vi "Navigation_Main_r1.5 (going back to derp).vi"() -> ()   [LabVIEW 2015]
uses:
  <vilib>/myRIO/Instrument Drivers/Onboard IO/PWM/typedefs/PWM Reference.ctl
  <vilib>/myRIO/Common/Instrument Driver Framework/Utilities/typedefs/myRIO Generic Hardware Reference.ctl
  <vilib>/myRIO/Common/Instrument Driver Framework/Utilities/typedefs/Hardware Version Enum.ctl
  <vilib>/myRIO/Common/Instrument Driver Framework/Utilities/typedefs/myRIO v1.0 Reference.ctl
  <vilib>/myRIO/Common/Instrument Driver Framework/Utilities/typedefs/Generic FPGA Reference.ctl
  <vilib>/myRIO/Common/Instrument Driver Framework/myRIO v1.0/PWM/typedefs/PWM Channels Enum.ctl
  <vilib>/myRIO/Instrument Drivers/Onboard IO/PWM/typedefs/PWM Configuration.ctl
  <vilib>/userdefined/High Color/nirio_resource_hc.ctl
  <vilib>/myRIO/Common/Instrument Driver Framework/myRIO v1.0/PWM/vis/myRIO v1.1 Open PWM.vi
  <vilib>/myRIO/Common/Instrument Driver Framework/Utilities/vis/Validate Channels.vi
  <vilib>/myRIO/Common/Instrument Driver Framework/myRIO v1.0/PWM/vis/myRIO v1.0 Reserve PWM.vi
  <vilib>/myRIO/Common/Instrument Driver Framework/myRIO v1.0/PWM/vis/myRIO v1.0 Close PWM.vi
  <vilib>/myRIO/Common/Instrument Driver Framework/myRIO v1.0/PWM/vis/myRIO v1.0 Build MUX Configuration PWM.vi
  <vilib>/myRIO/Common/Instrument Driver Framework/myRIO v1.0/Resource Manager/vis/myRIO v1.0 Reserve Channel List.vi
  <vilib>/myRIO/Common/Instrument Driver Framework/myRIO v1.0/PWM/vis/myRIO v1.0 Unreserve PWM.vi
  <vilib>/myRIO/Common/Instrument Driver Framework/myRIO v1.0/Resource Manager/vis/myRIO v1.0 Create Configuration List.vi
  <vilib>/myRIO/Common/Instrument Driver Framework/myRIO v1.0/Resource Manager/vis/myRIO v1.0 Reserve Channel.vi
  <vilib>/myRIO/Common/Instrument Driver Framework/myRIO v1.0/Resource Manager/vis/myRIO v1.0 Unreserve Channel.vi
  <vilib>/myRIO/Common/Instrument Driver Framework/myRIO v1.0/Resource Manager/vis/myRIO v1.0 Unreserve Channel List.vi
  <vilib>/myRIO/Common/Instrument Driver Framework/myRIO v1.0/Resource Manager/vis/myRIO v1.0 Build Mutex Name.vi
  <vilib>/FPGAPlugInAG/myRIO-1900/niLvFpga_Open_myRIO-1900.vi
  <vilib>/rvi/interface/common/dynamic/niFpgaDynamicAddResources.vi
  <vilib>/myRIO/Common/Instrument Driver Framework/Utilities/vis/FPGA Ref Manager.vi
  <vilib>/Utility/error.llb/Error Cluster From Error Code.vi
  <vilib>/myRIO/Common/Instrument Driver Framework/Utilities/vis/Ref Counter.vi
  <vilib>/rvi/errors/niLvFpgaAdjustHostInterfaceError.vi
  <vilib>/Utility/VariantDataType/GetNumericInfo.vi
  <vilib>/myRIO/Common/Instrument Driver Framework/myRIO v1.0/myRIO v1.1 Open.vi
  <vilib>/myRIO/Common/Instrument Driver Framework/Utilities/vis/IO Manager.vi
  <vilib>/myRIO/Common/Instrument Driver Framework/Utilities/vis/Configuration Manager.vi
  <vilib>/myRIO/Common/Instrument Driver Framework/myRIO v1.0/Resource Manager/vis/myRIO v1.0 Configure IO.vi
  <vilib>/myRIO/Common/Instrument Driver Framework/myRIO v1.0/myRIO v1.0 Close.vi
  <vilib>/myRIO/Common/Instrument Driver Framework/myRIO v1.0/PWM/vis/myRIO v1.0 Write PWM.vi
  <vilib>/myRIO/Common/Instrument Driver Framework/myRIO v1.0/PWM/vis/myRIO v1.0 Shutdown PWM.vi
  <vilib>/rvi/interface/nirviOpenFPGA/nirviOpenFPGA.xnode
  Navi/E/FPGA Bitfiles/NavigationProjec_FPGATarget2_FPGAMainNavigati_PWPHW8gwDxI.lvbitx
  <vilib>/rvi/interface/nirviReadWriteControl/nirviReadWriteControl.xnode
  <vilib>/myRIO/Instrument Drivers/Onboard IO/PWM/vis/myRIO PWM Open.xnode
  <vilib>/myRIO/Instrument Drivers/Onboard IO/PWM/PWM.lvlib
  <vilib>/myRIO/Instrument Drivers/Utilities/Utilities.lvlib
  NiFpgaLv.dll
  <vilib>/rvi/interface/Simulation/niFpgaSimulationCallBeginRW.vi
panel:
  out "cout per foot":dbl
  in  "start y 2":dbl=3.0
  in  "start x 2":dbl=1.0
  in  "Encoder Reset 2":bool
  out "x traveled 2":dbl
  out "y traveled 2":dbl
  out "avg right":dbl
  out "avg left":dbl
  out "psi dot 2":dbl
  out "distance traveled 2":dbl
  out "y dot 2":dbl
  out "x dot 2":dbl
  out "x position 2":dbl
  out "y position 2":dbl
  out "reset x y 2":dbl
  out "Tick Count(mSec) 2":u32 caption="Tick Count(mSec)"
  out "right":dbl
  out "left":dbl
  in  "start x":dbl=1.0
  in  "start y":dbl=3.0
  in  "x goal":dbl=10.0
  out "scale":dbl=1.0
  out "x/y":dbl
  in  "Goal Position Y":dbl=5.0
  out "track width(ft)":dbl=4.0
  out "RM Distance (ft)":dbl
  out "RR Distance (ft)":dbl
  out "LF Distance (ft)":dbl
  out "LM Distance (ft)":dbl
  out "RF Distance (ft)":dbl
  out "LR Distance (ft)":dbl
  in  "Start Position Y":dbl=5.0
  in  "Goal Position X":dbl=5.0
  in  "Start Position X":dbl=1.0
  in  "All Stop":bool
  in  "Left Side PID Gains":T1={"proportional gain (Kc)"=0.002, "integral time (Ti, min)"=7e-07, "derivative time (Td, min)"=0.0} {"derivative time (Td, min)" format="%.8f"; "integral time (Ti, min)" format="%.8f"; "proportional gain (Kc)" format="%.8f"}
  in  "Left Side Output Range":cluster{"output high":dbl, "output low":dbl}={"output high"=0.13333, "output low"=-0.13333} {"output low" format="%.5f"; "output high" format="%.5f"}
  in  "Right Side PID Gains":T1={"proportional gain (Kc)"=0.002, "integral time (Ti, min)"=7e-07, "derivative time (Td, min)"=0.0} {"derivative time (Td, min)" format="%.8f"; "integral time (Ti, min)" format="%.8f"; "proportional gain (Kc)" format="%.8f"}
  in  "Right Side Output Range":cluster{"output high":dbl, "output low":dbl}={"output high"=0.13333, "output low"=-0.13333} {"output low" format="%.5f"; "output high" format="%.5f"}
  out "Left PWM":dbl
  out "Right PWM":dbl
  out "LF Rot Velocity (rot/s)":dbl
  out "LM Rot Velocity (rot/s)":dbl
  out "LR Rot Velocity (rot/s)":dbl
  out "RR Rot Velocity (rot/s)":dbl
  out "RM Linear Velocity (rot/s)":dbl
  out "RF Linear Velocity (rot/s)":dbl
  in  "Encoder Reset":bool
  out "SYS.SELECTA":u8 format="%08b"
  out "ENC.B_c.CNTR":i32
  out "ENC.B_b.CNTR":i32
  out "ENC.B_a.CNTR":i32
  out "ENC.A_c.CNTR":i32
  out "ENC.A_b.CNTR":i32
  out "ENC.A_a.CNTR":i32
  out "Current Rot Velocity (rot/s)":T2(graph)
  # "Motor Control Parameters"
  # "Press Go when Start and Goal Are Set"
types:
  T1 = cluster{"proportional gain (Kc)":dbl, "integral time (Ti, min)":dbl, "derivative time (Td, min)":dbl}
  T2 = cluster{"Rotational Velocity (RPS)":dbl, "Rotational Velocity (RPS)":dbl, "Rotational Velocity (RPS)":dbl, "Rotational Velocity (RPS)":dbl, "Rotational Velocity (RPS)":dbl, "Rotational Velocity (RPS)":dbl}
  T3 = typedef "nirio_resource_hc.ctl" = tag
  T4 = typedef "Hardware Version Enum.ctl" = enum16{"Unknown", "myRIO-1900", "myRIO-1950", "roboRIO"}
  T5 = typedef "PWM.lvlib/PWM Reference.ctl" = cluster{"myRIO Reference":T6, "PWM Channels Enum":T9, "PWM Configuration":T10}
  T6 = typedef "myRIO Generic Hardware Reference.ctl" = cluster{"myRIO Model":T4, "myRIO Hardware Reference":T7}
  T7 = typedef "myRIO v1.0 Reference.ctl" = cluster{"Generic FPGA Reference":T8, "Allow multiple opens":bool}
  T8 = typedef "Generic FPGA Reference.ctl" = refnum<k20>
  T9 = typedef "PWM Channels Enum.ctl" = enum16{"Not Connected", "C/PWM0", "C/PWM1", "A/PWM0", "A/PWM1", "A/PWM2", "B/PWM0", "B/PWM1", "B/PWM2", "PWM/PWM0", "PWM/PWM1", "PWM/PWM2", "PWM/PWM3", "PWM/PWM4", "PWM/PWM5", "PWM/PWM6", "PWM/PWM7", "PWM/PWM8", "PWM/PWM9"}
  T10 = typedef "PWM.lvlib/PWM Configuration.ctl" = cluster{"Frequency":dbl, "Duty Cycle":dbl}
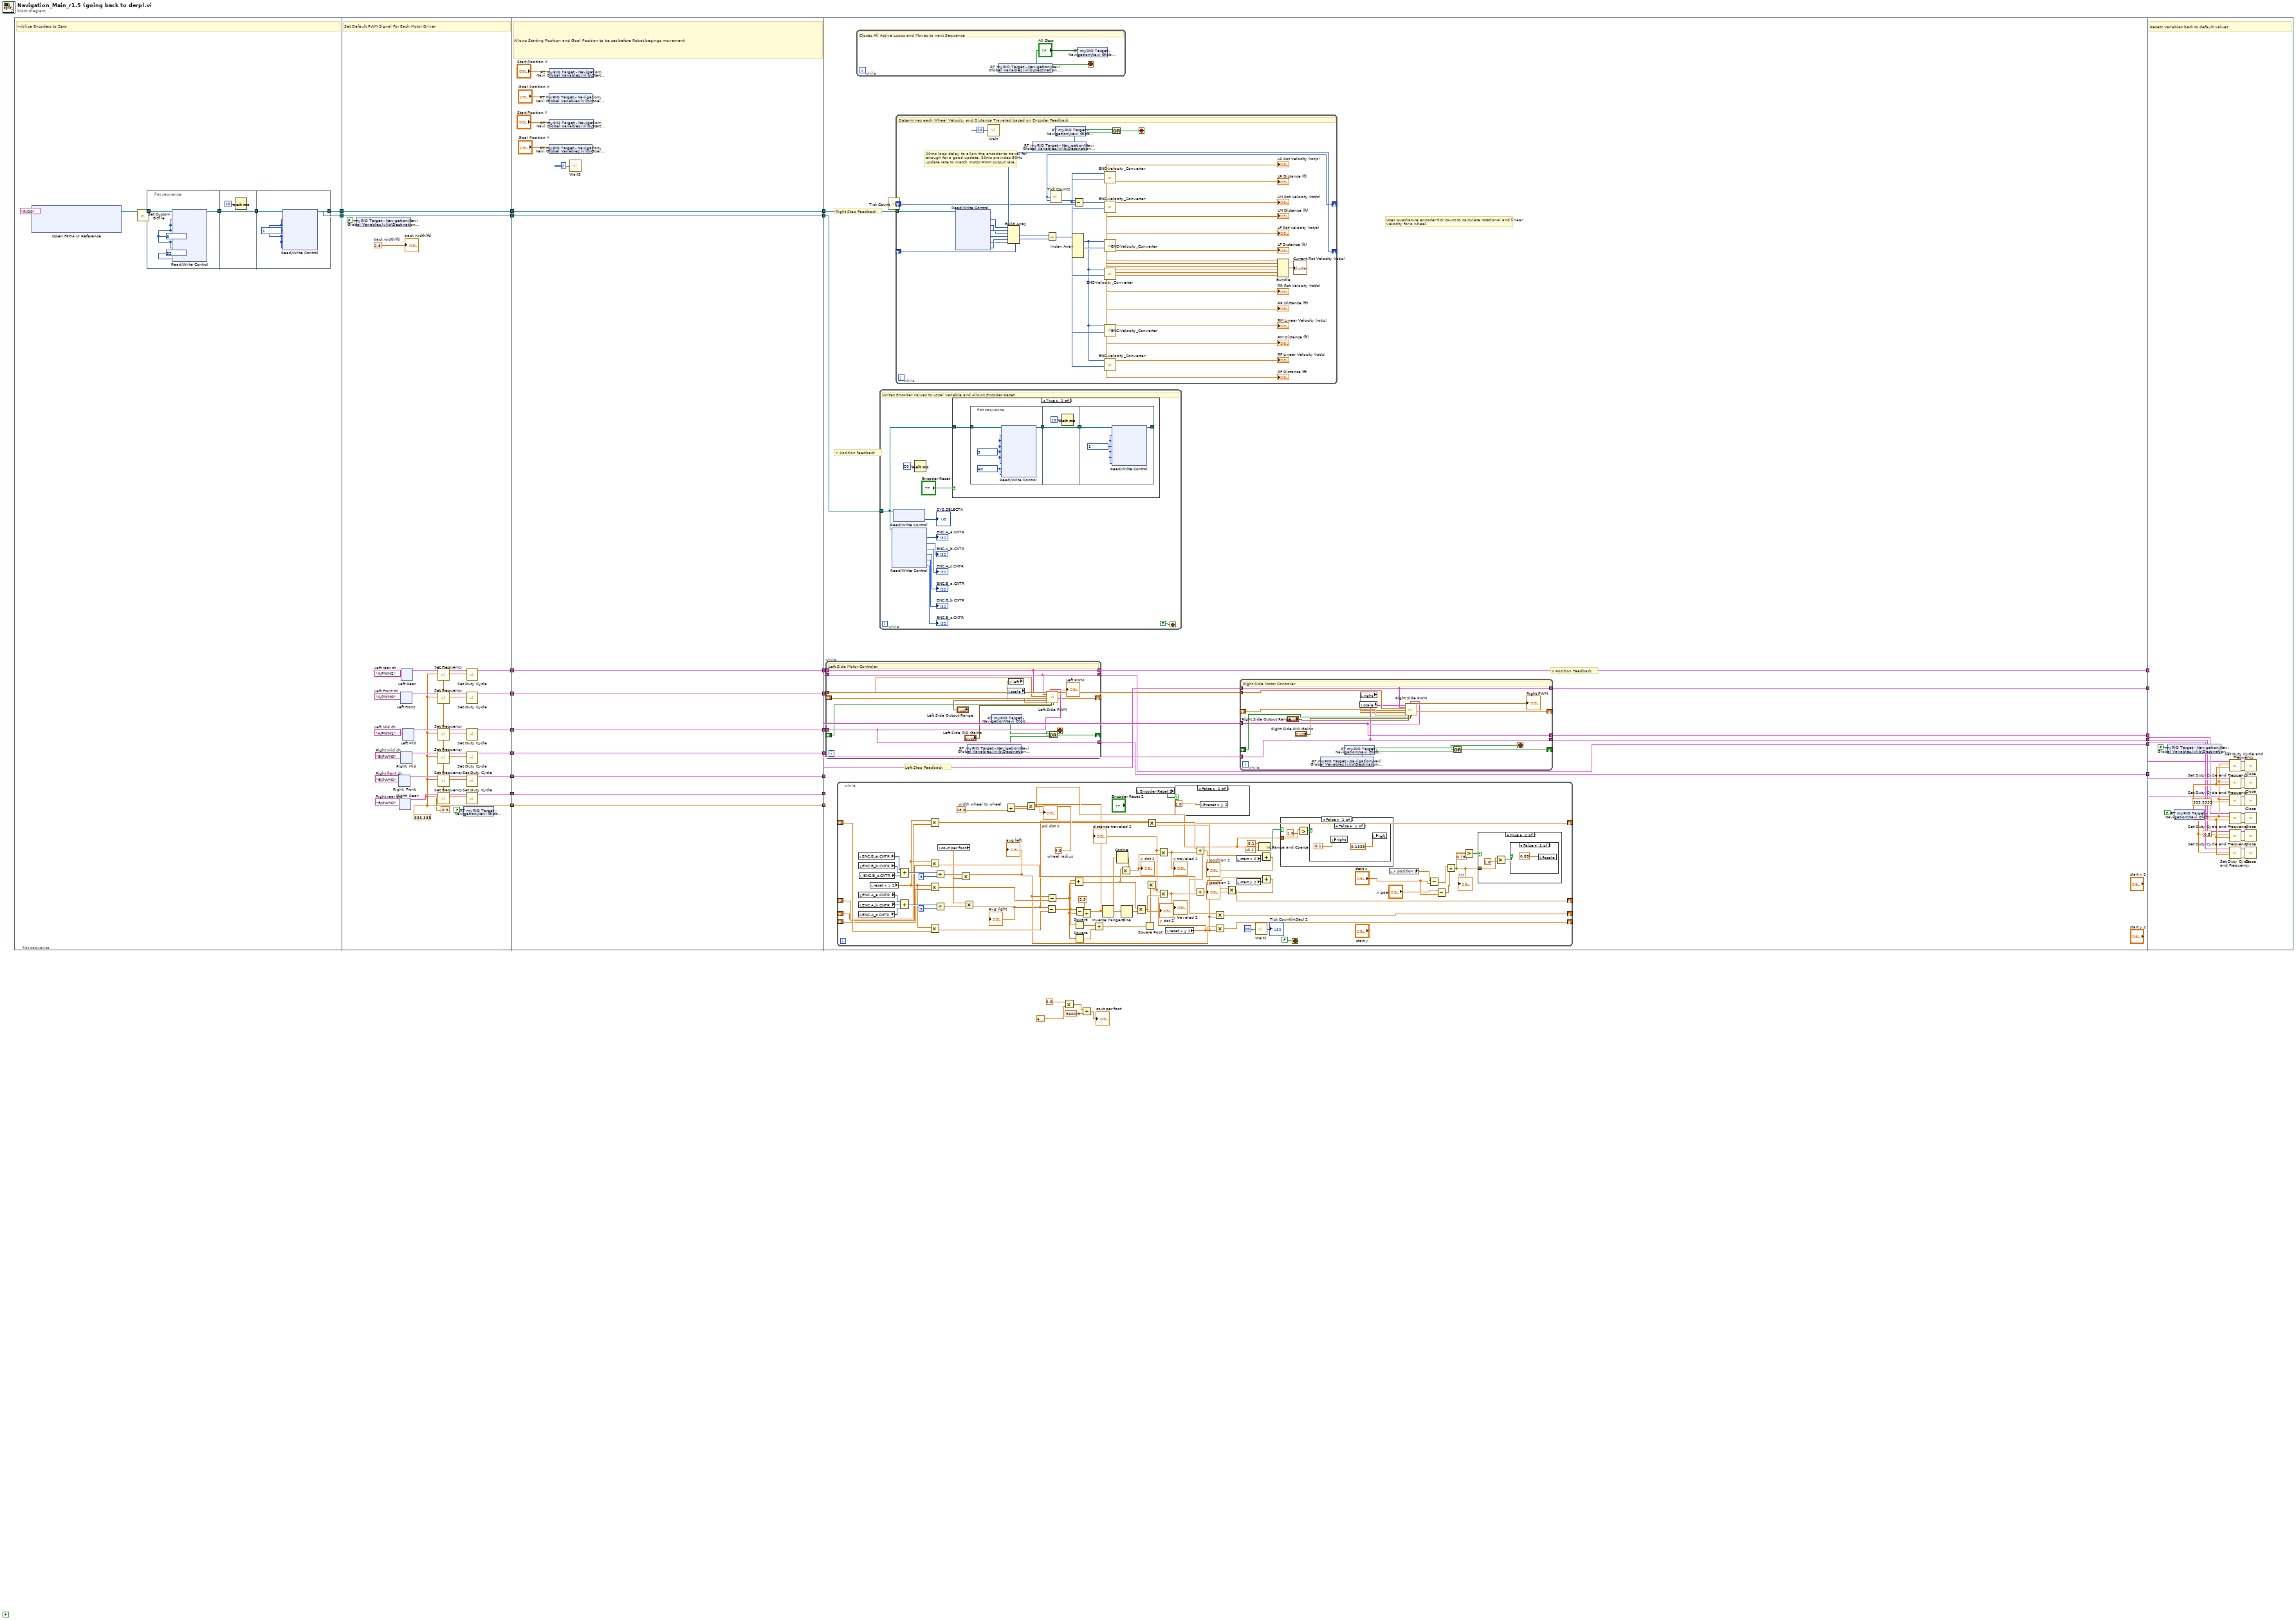
[diagram p0: block diagram]
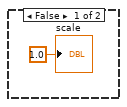
[diagram p2: hidden frame]
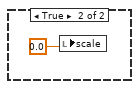
[diagram p3: hidden frame]
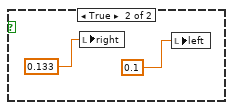
[diagram p4: hidden frame]
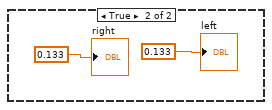
[diagram p5: hidden frame]
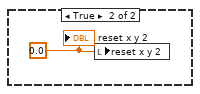
[diagram p6: hidden frame]
diagram:
  (unwired) FALSE ("stop")
  n1 = flat-sequence {
    tunnel: [w34] -> w31
    tunnel: [w34] -> w30
    tunnel: [w65] -> w29
    tunnel: [w60] -> w28
    tunnel: [w56] -> w27
    tunnel: [w55] -> w26
    tunnel: [w54] -> w25
    tunnel: [w53] -> w24
    tunnel: [w52] -> w23
    tunnel: [w51] -> w22
    tunnel: w31 -> [w50]
    tunnel: [w50] -> w21
    tunnel: w30 -> [w51]
    tunnel: w29 -> [w187]
    tunnel: [w187] -> w20
    tunnel: w28 -> [w186]
    tunnel: [w186] -> w19
    tunnel: w27 -> [w185]
    tunnel: [w185] -> w18
    tunnel: w26 -> [w174]
    tunnel: [w174] -> w17
    tunnel: w25 -> [w184]
    tunnel: [w184] -> w16
    tunnel: w24 -> [w183]
    tunnel: [w183] -> w15
    tunnel: w23 -> [w182]
    tunnel: [w182] -> w14
    tunnel: w22 -> [w181]
    tunnel: [w181] -> w13
    tunnel: w21 -> [w180]
    tunnel: [w180] -> w12
    tunnel: w20 -> [w194]
    tunnel: w19 -> [w195]
    tunnel: w18 -> [w200]
    tunnel: w17 -> [w199]
    tunnel: w16 -> [w198]
    tunnel: w15 -> [w197]
    tunnel: w14 -> [w196]
    tunnel: w13 -> [w202]
    tunnel: w12 -> [w201]
    tunnel: [w193] -> w11
    tunnel: [w192] -> w10
    tunnel: [w191] -> w9
    tunnel: [w190] -> w8
    tunnel: [w189] -> w7
    tunnel: [w188] -> w6
    tunnel: w11 -> [w390]
    tunnel: w10 -> [w389]
    tunnel: w9 -> [w388]
    tunnel: w8 -> [w387]
    tunnel: w7 -> [w386]
    tunnel: w6 -> [w385]
    frame #0 {
      # "Initilize Encoders to Zero"
      n2 = xnode "Open FPGA VI Reference"("resource name"=tag "RIO0") -> ("FPGA VI Reference Out"=w33:refnum<k20>)  [unwired: 1 in, 1 out]
      n3 = call <vilib>:"Set Custom Bitfile.vi"("Custom FPGA Reference In"=w33) -> ("Custom FPGA Reference Out"=w35:refnum<k20>)  [unwired: 9 in, 1 out]
      n4 = flat-sequence {
        tunnel: w35 -> [w40]
        tunnel: [w38] -> w37
        tunnel: w37 -> [w42]
        tunnel: [w42] -> w36
        tunnel: w36 -> [w45]
        tunnel: [w44] -> w34
        frame #0 {
          w39 = u8 32 ("SYS.SELECTA")
          w41 = u8 3 ("ENC.B_c.CNFG")
          n5 = xnode "Read/Write Control"("FPGA VI Reference In"=w40, "ENC.A_a.CNFG"=w41, "ENC.A_b.CNFG"=w41, "ENC.A_c.CNFG"=w41, "ENC.B_a.CNFG"=w41, "ENC.B_b.CNFG"=w41, "ENC.B_c.CNFG"=w41, "SYS.SELECTA"=w39, "SYS.SELECTB"=w39) -> ("FPGA VI Reference Out"=w38:refnum<k20>)  [unwired: 1 in, 1 out]
        }
        frame #1 {
          n6 = Wait (ms)(milliseconds to wait=u32 10) -> ()  [unwired: 1 out]
        }
        frame #2 {
          w46 = u8 1 ("ENC.B_c.CNFG")
          n7 = xnode "Read/Write Control"("FPGA VI Reference In"=w45, "ENC.A_a.CNFG"=w46, "ENC.A_b.CNFG"=w46, "ENC.A_c.CNFG"=w46, "ENC.B_a.CNFG"=w46, "ENC.B_b.CNFG"=w46, "ENC.B_c.CNFG"=w46) -> ("FPGA VI Reference Out"=w44:refnum<k20>)  [unwired: 1 in, 1 out]
        }
      }
    }
    frame #1 {
      w47 = 2.5  # track width(ft)
      w57 = 0.5 ("Duty Cycle")
      w65 = 333.333 ("Frequency [Hz]")
      w72 = tag "B/PWM2"  # Right rear ch
      w73 = tag "B/PWM0"  # Right mid ch
      w74 = tag "B/PWM1"  # Right front ch
      w75 = tag "A/PWM2"  # Left rear ch
      w76 = tag "A/PWM0"  # Left Front ch
      w77 = tag "A/PWM1"  # Left Mid ch
      # "Set Default PWM Signal For Each Motor Driver"
      n8 = shared-variable "RT myRIO Target - Navigation\\Navi Global Variables.lvlib\\Destination Reached"(FALSE) -> ()  [unwired: 1 in, 1 out]
      n9 = xnode "Right  Front"("Channel Name"=w74) -> ("PWM Ref Out"=w68:T5)  [unwired: 2 in, 1 out]
      n10 = xnode "Right  Rear"("Channel Name"=w72) -> ("PWM Ref Out"=w66:T5)  [unwired: 2 in, 1 out]
      n11 = xnode "Left Front"("Channel Name"=w76) -> ("PWM Ref Out"=w70:T5)  [unwired: 2 in, 1 out]
      n12 = xnode "Right  Mid"("Channel Name"=w73) -> ("PWM Ref Out"=w67:T5)  [unwired: 2 in, 1 out]
      n13 = xnode "Left Rear"("Channel Name"=w75) -> ("PWM Ref Out"=w69:T5)  [unwired: 2 in, 1 out]
      n14 = xnode "Left Mid"("Channel Name"=w77) -> ("PWM Ref Out"=w71:T5)  [unwired: 2 in, 1 out]
      n15 = call <vilib>:"Set Frequency.vi"("Frequency [Hz]"=w65, "PWM Ref In"=w69) -> ("PWM Ref Out"=w59:T5)  [unwired: 7 in, 1 out]
      n16 = call <vilib>:"Set Frequency.vi"("Frequency [Hz]"=w65, "PWM Ref In"=w70) -> ("PWM Ref Out"=w58:T5)  [unwired: 7 in, 1 out]
      n17 = call <vilib>:"Set Frequency.vi"("Frequency [Hz]"=w65, "PWM Ref In"=w71) -> ("PWM Ref Out"=w64:T5)  [unwired: 7 in, 1 out]
      n18 = call <vilib>:"Set Frequency.vi"("Frequency [Hz]"=w65, "PWM Ref In"=w67) -> ("PWM Ref Out"=w62:T5)  [unwired: 7 in, 1 out]
      n19 = call <vilib>:"Set Frequency.vi"("Frequency [Hz]"=w65, "PWM Ref In"=w68) -> ("PWM Ref Out"=w61:T5)  [unwired: 7 in, 1 out]
      n20 = call <vilib>:"Set Frequency.vi"("Frequency [Hz]"=w65, "PWM Ref In"=w66) -> ("PWM Ref Out"=w63:T5)  [unwired: 7 in, 1 out]
      n21 = shared-variable "RT myRIO Target - Navigation\\Navi Global Variables.lvlib\\All Stop"(FALSE) -> ()  [unwired: 1 in, 1 out]
      n22 = call <vilib>:"Set Duty Cycle.vi"("Duty Cycle"=w57, "PWM Ref In"=w59) -> ("PWM Ref Out"=w60:T5)  [unwired: 7 in, 1 out]
      n23 = call <vilib>:"Set Duty Cycle.vi"("Duty Cycle"=w57, "PWM Ref In"=w58) -> ("PWM Ref Out"=w53:T5)  [unwired: 7 in, 1 out]
      n24 = call <vilib>:"Set Duty Cycle.vi"("Duty Cycle"=w57, "PWM Ref In"=w64) -> ("PWM Ref Out"=w52:T5)  [unwired: 7 in, 1 out]
      n25 = call <vilib>:"Set Duty Cycle.vi"("Duty Cycle"=w57, "PWM Ref In"=w62) -> ("PWM Ref Out"=w55:T5)  [unwired: 7 in, 1 out]
      n26 = call <vilib>:"Set Duty Cycle.vi"("Duty Cycle"=w57, "PWM Ref In"=w61) -> ("PWM Ref Out"=w56:T5)  [unwired: 7 in, 1 out]
      n27 = call <vilib>:"Set Duty Cycle.vi"("Duty Cycle"=w57, "PWM Ref In"=w63) -> ("PWM Ref Out"=w54:T5)  [unwired: 7 in, 1 out]
      "track width(ft)" <- w47
    }
    frame #2 {
      # "Allows Starting Position and Goal Position to be set before Robot begings movement"
      n28 = shared-variable "RT myRIO Target - Navigation\\Navi Global Variables.lvlib\\Start Position X"("Start Position X") -> ()  [unwired: 1 in, 1 out]
      n29 = shared-variable "RT myRIO Target - Navigation\\Navi Global Variables.lvlib\\Goal Position X"("Goal Position X") -> ()  [unwired: 1 in, 1 out]
      n30 = shared-variable "RT myRIO Target - Navigation\\Navi Global Variables.lvlib\\Start Position Y"("Start Position Y") -> ()  [unwired: 1 in, 1 out]
      n31 = shared-variable "RT myRIO Target - Navigation\\Navi Global Variables.lvlib\\Goal Position Y"("Goal Position Y") -> ()  [unwired: 1 in, 1 out]
      n32 = call "Wait3"("Count(mSec)"=u32 2) -> ()  [unwired: 1 out]
    }
    frame #3 {
      # "Left Step Feedback"
      # "Y Position feedback"
      # "Right Step Feedback"
      # "X Position Feedback"
      # "Uses quadrature encoder tick count to calculate rotational and linear velocity for a wheel."
      n33 = while {
        tunnel: w197 -> [w301]
        tunnel: w196 -> [w300]
        tunnel: w195 -> [w299]
        tunnel: w194 -> [w308]
        shift-right: [w304] -> _
        shift-left: _ -> [w303]
        shift-right: [w296] -> _
        shift-left: _ -> [w302]
        tunnel: [w301] -> w190
        tunnel: [w300] -> w189
        tunnel: [w299] -> w188
        stop <- w296 stop-if-true
        # "Left Side Motor Controler"
        n34 = shared-variable "RT myRIO Target - Navigation\\Navi Global Variables.lvlib\\Destination Reached"() -> (w298:bool)  [unwired: 1 in, 1 out]
        n35 = shared-variable "RT myRIO Target - Navigation\\Navi Global Variables.lvlib\\All Stop"() -> (w297:bool)  [unwired: 1 in, 1 out]
        n36 = local read "scale"() -> (w294:dbl)
        n37 = local read "left"() -> (w295:dbl)
        n38 = call "Left Side PWM.vi"("Left rear"=w299, "Frequency"=w308, "Left Side Setpoint"=w295, "Left Side Scale"=w294, "Left PID Feedback"=w303, "Left Mid"=w300, "Left Side Output Range"="Left Side Output Range", "Left Front"=w301, "Left Side PID Gains"="Left Side PID Gains", "Reset Left E.T."=w302) -> ("Left PWM"=→"Left PWM":dbl, "Left PID Output"=w304:dbl)  [unwired: 8 in]
        n39 = Or(x=w297, y=w298) -> (x .or. y?=w296:bool)
      }
      n40 = while {
        shift-right: [w232] -> _
        shift-left: _ -> [w262]
        shift-right: [w229] -> _
        shift-left: _ -> [w261]
        shift-right: [w231] -> _
        shift-left: _ -> [w241]
        shift-right: [w230] -> _
        shift-left: _ -> [w240]
        stop <- FALSE stop-if-true
        w258 = 28.0  # width wheel to wheel
        w259 = 4.0  # wheel radius
        n41 = local read "ENC.B_a.CNTR"() -> (w267:i32)
        n42 = local read "ENC.B_b.CNTR"() -> (w266:i32)
        n43 = local read "ENC.A_a.CNTR"() -> (w270:i32)
        n44 = local read "ENC.A_b.CNTR"() -> (w269:i32)
        n45 = local read "ENC.A_c.CNTR"() -> (w268:i32)
        n46 = local read "ENC.B_c.CNTR"() -> (w265:i32)
        n47 = local read "reset x y 2"() -> (w228:dbl)
        n48 = Compound Arithmetic op=ADD(w267, w266, w265) -> (w273:i32)
        n49 = Compound Arithmetic op=ADD(w270, w269, w268) -> (w274:i32)
        n50 = Multiply(x=w228, y=w240) -> (x*y=w234:dbl)
        n51 = Multiply(x=w228, y=w241) -> (x*y=w235:dbl)
        n52 = Multiply(x=w228, y=w261) -> (x*y=w233:dbl)
        n53 = Multiply(x=w228, y=w262) -> (x*y=w236:dbl)
        n54 = Divide(x=w273, y=3) -> (x/y=w260:dbl)
        n55 = Divide(x=w274, y=3) -> (x/y=w263:dbl)
        n56 = local read "cout per foot"() -> (w207:dbl)
        n57 = Multiply(x=w260, y=w207) -> (x*y=w209:dbl)
        "avg left" <- w209
        n58 = Multiply(x=w207, y=w263) -> (x*y=w208:dbl)
        "avg right" <- w208
        n59 = Divide(x=w259, y=w258) -> (x/y=w255:dbl)
        n60 = Subtract(x=w208, y=w236) -> (x-y=w204:dbl)
        n61 = Subtract(x=w209, y=w233) -> (x-y=w253:dbl)
        n62 = Add(x=w204, y=w253) -> (x+y=w257:dbl)
        n63 = Square(x=w204) -> (x^2=w251:dbl)
        n64 = Square(x=w253) -> (x^2=w252:dbl)
        n65 = Subtract(x=w204, y=w253) -> (x-y=w256:dbl)
        n66 = Divide(x=w256, y=2.5) -> (x/y=w206:dbl)
        n67 = Multiply(x=w206, y=w255) -> (x*y=w218:dbl)
        "psi dot 2" <- w218
        n68 = Add(x=w251, y=w252) -> (x+y=w250:dbl)
        n69 = Inverse Tangent(1:w206) -> (0:w254:dbl)
        n70 = Cosine(x=w254) -> (cos(x)=w248:dbl)
        n71 = Multiply(x=w257, y=w248) -> (x*y=w246:dbl)
        "x dot 2" <- w246
        n72 = Sine(x=w254) -> (sin(x)=w249:dbl)
        n73 = Multiply(x=w257, y=w249) -> (x*y=w247:dbl)
        "y dot 2" <- w247
        n74 = local read "Encoder Reset 2"() -> (w225:bool)
        n75 = Square Root(x=w250) -> (sqrt(x)=w245:dbl)
        n76 = local read "reset x y 2"() -> (w226:dbl)
        n77 = Multiply(x=w245, y=w226) -> (x*y=w227:dbl)
        "distance traveled 2" <- w227
        n78 = Multiply(x=w208, y=w226) -> (x*y=w232:dbl)
        n79 = Multiply(x=w227, y=w246) -> (x*y=w244:dbl)
        "x traveled 2" <- w244
        n80 = Multiply(x=w227, y=w247) -> (x*y=w243:dbl)
        "y traveled 2" <- w243
        n81 = case shown="False" w225 {
          frame False {
            n82 = local write "reset x y 2"(1.0) -> ()
          }
          frame True {
            w292 = 0.0
            n83 = local write "reset x y 2"(w292) -> ()
            "reset x y 2" <- w292
          }
        }
        n84 = Add(x=w234, y=w244) -> (x+y=w242:dbl)
        n85 = Add(x=w235, y=w243) -> (x+y=w237:dbl)
        n86 = Multiply(x=w242, y=w226) -> (x*y=w230:dbl)
        n87 = Multiply(x=w209, y=w226) -> (x*y=w229:dbl)
        n88 = Multiply(x=w226, y=w237) -> (x*y=w231:dbl)
        n89 = local read "start x 2"() -> (w238:dbl)
        n90 = local read "start y 2"() -> (w239:dbl)
        n91 = call "Wait2"("Count(mSec)"=u32 20) -> ("Tick Count(mSec)"=→"Tick Count(mSec) 2":u32)
        n92 = In Range and Coerce(upper limit=0.1, x=w218, lower limit=-0.1) -> (In Range?=w219:bool)  [unwired: 1 out]
        n93 = Add(x=w242, y=w238) -> (x+y=→"x position 2":dbl)
        n94 = Add(x=w237, y=w239) -> (x+y=→"y position 2":dbl)
        n95 = case shown="False" w219 {
          tunnel: w218 -> [w284 _]
          frame False {
            n96 = Greater?(x=w284, y=1.0) -> (0:w282:bool)
            n97 = case shown="False" w282 {
              frame False {
                n98 = local write "right"(0.1) -> ()
                n99 = local write "left"(0.1333) -> ()
              }
              frame True {
                n100 = local write "right"(0.133) -> ()
                n101 = local write "left"(0.1) -> ()
              }
            }
          }
          frame True {
            "right" <- 0.133
            "left" <- 0.133
          }
        }
        n102 = local read "x position 2"() -> (w217:dbl)
        n103 = Subtract(x=w217, y="start x") -> (x-y=w211:dbl)
        n104 = Subtract(x="x goal", y="start x") -> (x-y=w210:dbl)
        n105 = Divide(x=w211, y=w210) -> (x/y=w214:dbl)
        "x/y" <- w214
        n106 = Greater?(x=w214, y=0.75) -> (0:w215:bool)
        n107 = case shown="True" w215 {
          tunnel: w214 -> [_ w279]
          frame False {
            "scale" <- 1.0
          }
          frame True {
            n108 = Greater?(x=w279, y=1.0) -> (0:w277:bool)
            n109 = case shown="False" w277 {
              frame False {
                n110 = local write "scale"(0.85) -> ()
              }
              frame True {
                n111 = local write "scale"(0.0) -> ()
              }
            }
          }
        }
      }
      n112 = while {
        stop <- "All Stop" stop-if-true
        # "Closes All Active Loops and Moves to next Sequence"
        n113 = shared-variable "RT myRIO Target - Navigation\\Navi Global Variables.lvlib\\Destination Reached"() -> ()  [unwired: 1 in, 2 out]
        n114 = shared-variable "RT myRIO Target - Navigation\\Navi Global Variables.lvlib\\All Stop"("All Stop") -> ()  [unwired: 1 in, 1 out]
      }
      n115 = while {
        tunnel: w202 -> [w325]
        stop <- FALSE stop-if-true
        # "Writes Encoder Values to Local Variable and Allows Encoder Reset"
        n116 = xnode "Read/Write Control"("FPGA VI Reference In"=w325) -> ("ENC.A_a.CNTR"=→"ENC.A_a.CNTR":u32, "ENC.A_b.CNTR"=→"ENC.A_b.CNTR":u32, "ENC.A_c.CNTR"=→"ENC.A_c.CNTR":u32, "ENC.B_a.CNTR"=→"ENC.B_a.CNTR":u32, "ENC.B_b.CNTR"=→"ENC.B_b.CNTR":u32, "ENC.B_c.CNTR"=→"ENC.B_c.CNTR":u32)  [unwired: 1 in, 2 out]
        n117 = xnode "Read/Write Control"("FPGA VI Reference In"=w325) -> ("SYS.SELECTA"=→"SYS.SELECTA":u8)  [unwired: 1 in, 2 out]
        n118 = Wait (ms)(milliseconds to wait=u32 20) -> ()  [unwired: 1 out]
        n119 = case shown="True" "Encoder Reset" {
          tunnel: w325 -> [_ w335]
          frame False {
          }
          frame True {
            n120 = flat-sequence {
              tunnel: w335 -> [w340]
              tunnel: [w338] -> w337
              tunnel: w337 -> [w342]
              tunnel: [w342] -> w336
              tunnel: w336 -> [w345]
              tunnel: [w344] -> _
              frame #0 {
                w339 = u8 60 ("SYS.SELECTA")
                w341 = u8 3 ("ENC.B_c.CNFG")
                n121 = xnode "Read/Write Control"("FPGA VI Reference In"=w340, "ENC.A_a.CNFG"=w341, "ENC.A_b.CNFG"=w341, "ENC.A_c.CNFG"=w341, "ENC.B_a.CNFG"=w341, "ENC.B_b.CNFG"=w341, "ENC.B_c.CNFG"=w341, "SYS.SELECTA"=w339, "SYS.SELECTB"=w339) -> ("FPGA VI Reference Out"=w338:refnum<k20>)  [unwired: 1 in, 1 out]
              }
              frame #1 {
                n122 = Wait (ms)(milliseconds to wait=u32 10) -> ()  [unwired: 1 out]
              }
              frame #2 {
                w346 = u8 1 ("ENC.B_c.CNFG")
                n123 = xnode "Read/Write Control"("FPGA VI Reference In"=w345, "ENC.A_a.CNFG"=w346, "ENC.A_b.CNFG"=w346, "ENC.A_c.CNFG"=w346, "ENC.B_a.CNFG"=w346, "ENC.B_b.CNFG"=w346, "ENC.B_c.CNFG"=w346) -> ("FPGA VI Reference Out"=w344:refnum<k20>)  [unwired: 1 in, 1 out]
              }
            }
          }
        }
      }
      n124 = call "Tick Count"() -> ("Tick Count(uSec)"=w203:u32)
      n125 = while {
        shift-right: [w374] -> _
        shift-left: _ -> [w373]
        shift-right: [w371] -> _
        shift-left: w203 -> [w370]
        tunnel: w201 -> [w381]
        stop <- w366 stop-if-true
        # "20ms loop delay to allow the encoder to travel far enough for a good update. 20ms provides 50Hz update rate to match motor PWM output rate."
        # "Determines each Wheel Velocity and Distance Traveled based on Encoder Feedback"
        n126 = xnode "Read/Write Control"("FPGA VI Reference In"=w381) -> ("ENC.A_a.CNTR"=w380:u32, "ENC.A_b.CNTR"=w379:u32, "ENC.A_c.CNTR"=w378:u32, "ENC.B_a.CNTR"=w377:u32, "ENC.B_b.CNTR"=w376:u32, "ENC.B_c.CNTR"=w375:u32)  [unwired: 1 in, 2 out]
        n127 = call "Wait"("Count(mSec)"=u32 20) -> ()  [unwired: 1 out]
        n128 = Build Array(w380, w379, w378, w377, w376, w375) -> (w374:u32[])
        n129 = shared-variable "RT myRIO Target - Navigation\\Navi Global Variables.lvlib\\Destination Reached"() -> (w368:bool)  [unwired: 1 in, 1 out]
        n130 = Subtract(x=w374, y=w373) -> (x-y=w372:u32[])
        n131 = call "Tick Count2"() -> ("Tick Count(uSec)"=w371:u32)
        n132 = shared-variable "RT myRIO Target - Navigation\\Navi Global Variables.lvlib\\All Stop"() -> (w367:bool)  [unwired: 1 in, 1 out]
        n133 = Index Array(array=w372) -> (element #1=w365:u32, element #2=w362:u32, element #3=w360:u32, element #4=w358:u32, element #5=w356:u32, element #6=w353:u32)  [unwired: 6 in]
        n134 = Subtract(x=w371, y=w370) -> (x-y=w354:u32)
        n135 = call "ENC-Velocity_Converter.vi"("delta  Encoder Count"=w365, "dt (uSec)"=w354) -> ("Distance (ft)"=→"LR Distance (ft)":dbl, "Rotational Velocity (RPS)"=w364:dbl)  [unwired: 7 in, 1 out]
        "LR Rot Velocity (rot/s)" <- w364
        n136 = call "ENC-Velocity_Converter.vi"("delta  Encoder Count"=w362, "dt (uSec)"=w354) -> ("Distance (ft)"=→"LM Distance (ft)":dbl, "Rotational Velocity (RPS)"=w363:dbl)  [unwired: 7 in, 1 out]
        "LM Rot Velocity (rot/s)" <- w363
        n137 = call "ENC-Velocity_Converter.vi"("delta  Encoder Count"=w360, "dt (uSec)"=w354) -> ("Distance (ft)"=→"LF Distance (ft)":dbl, "Rotational Velocity (RPS)"=w361:dbl)  [unwired: 7 in, 1 out]
        "LF Rot Velocity (rot/s)" <- w361
        n138 = call "ENC-Velocity_Converter.vi"("delta  Encoder Count"=w358, "dt (uSec)"=w354) -> ("Distance (ft)"=→"RR Distance (ft)":dbl, "Rotational Velocity (RPS)"=w359:dbl)  [unwired: 7 in, 1 out]
        "RR Rot Velocity (rot/s)" <- w359
        n139 = call "ENC-Velocity_Converter.vi"("delta  Encoder Count"=w356, "dt (uSec)"=w354) -> ("Distance (ft)"=→"RM Distance (ft)":dbl, "Rotational Velocity (RPS)"=w357:dbl)  [unwired: 7 in, 1 out]
        "RM Linear Velocity (rot/s)" <- w357
        n140 = call "ENC-Velocity_Converter.vi"("delta  Encoder Count"=w353, "dt (uSec)"=w354) -> ("Distance (ft)"=→"RF Distance (ft)":dbl, "Rotational Velocity (RPS)"=w355:dbl)  [unwired: 7 in, 1 out]
        "RF Linear Velocity (rot/s)" <- w355
        n141 = Or(x=w367, y=w368) -> (x .or. y?=w366:bool)
        n142 = Bundle("Rotational Velocity (RPS)"=w364, "Rotational Velocity (RPS)"=w363, "Rotational Velocity (RPS)"=w361, "Rotational Velocity (RPS)"=w359, "Rotational Velocity (RPS)"=w357, "Rotational Velocity (RPS)"=w355) -> (→"Current Rot Velocity (rot/s)":T2)  [unwired: 1 in]
      }
      n143 = while {
        tunnel: w200 -> [w316]
        tunnel: w199 -> [w315]
        tunnel: w198 -> [w314]
        tunnel: w194 -> [w323]
        shift-right: [w319] -> _
        shift-left: _ -> [w318]
        shift-right: [w311] -> _
        shift-left: _ -> [w317]
        tunnel: [w316] -> w193
        tunnel: [w315] -> w192
        tunnel: [w314] -> w191
        stop <- w311 stop-if-true
        # "Right Side Motor Controler"
        n144 = shared-variable "RT myRIO Target - Navigation\\Navi Global Variables.lvlib\\Destination Reached"() -> (w313:bool)  [unwired: 1 in, 1 out]
        n145 = shared-variable "RT myRIO Target - Navigation\\Navi Global Variables.lvlib\\All Stop"() -> (w312:bool)  [unwired: 1 in, 1 out]
        n146 = local read "scale"() -> (w309:dbl)
        n147 = local read "right"() -> (w310:dbl)
        n148 = call "Right Side PWM.vi"("Right rear"=w314, "Frequency"=w323, "Right Side Setpoint"=w310, "Right Side Scale"=w309, "Right PID Feedback"=w318, "Right Mid"=w315, "Right Side Output Range"="Right Side Output Range", "Right Front"=w316, "Right Side PID Gains"="Right Side PID Gains", "Reset Right E.T."=w317) -> ("Right PWM"=→"Right PWM":dbl, "Right PID Output"=w319:dbl)  [unwired: 8 in]
        n149 = Or(x=w312, y=w313) -> (x .or. y?=w311:bool)
      }
    }
    frame #4 {
      w391 = 0.5
      w392 = 333.3333
      # "Resets Variables back to default values"
      n150 = shared-variable "RT myRIO Target - Navigation\\Navi Global Variables.lvlib\\Destination Reached"(FALSE) -> ()  [unwired: 1 in, 1 out]
      n151 = shared-variable "RT myRIO Target - Navigation\\Navi Global Variables.lvlib\\All Stop"(FALSE) -> ()  [unwired: 1 in, 1 out]
      n152 = call <vilib>:"Set Duty Cycle and Frequency.vi"("Frequency [Hz]"=w392, "Duty Cycle"=w391, "PWM Ref In"=w385) -> ("error out"=w393:errorcluster, "PWM Ref Out"=w398:T5)  [unwired: 6 in]
      n153 = call <vilib>:"Set Duty Cycle and Frequency.vi"("Frequency [Hz]"=w392, "Duty Cycle"=w391, "PWM Ref In"=w389) -> ("error out"=w402:errorcluster, "PWM Ref Out"=w403:T5)  [unwired: 6 in]
      n154 = call <vilib>:"Set Duty Cycle and Frequency.vi"("Frequency [Hz]"=w392, "Duty Cycle"=w391, "PWM Ref In"=w390) -> ("error out"=w397:errorcluster, "PWM Ref Out"=w404:T5)  [unwired: 6 in]
      n155 = call <vilib>:"Set Duty Cycle and Frequency.vi"("Frequency [Hz]"=w392, "Duty Cycle"=w391, "PWM Ref In"=w388) -> ("error out"=w396:errorcluster, "PWM Ref Out"=w401:T5)  [unwired: 6 in]
      n156 = call <vilib>:"Set Duty Cycle and Frequency.vi"("Frequency [Hz]"=w392, "Duty Cycle"=w391, "PWM Ref In"=w387) -> ("error out"=w395:errorcluster, "PWM Ref Out"=w400:T5)  [unwired: 6 in]
      n157 = call <vilib>:"Set Duty Cycle and Frequency.vi"("Frequency [Hz]"=w392, "Duty Cycle"=w391, "PWM Ref In"=w386) -> ("error out"=w394:errorcluster, "PWM Ref Out"=w399:T5)  [unwired: 6 in]
      n158 = call <vilib>:"Close.vi"("error in (no error)"=w393, "PWM Ref In"=w398) -> ()  [unwired: 9 in, 1 out]
      n159 = call <vilib>:"Close.vi"("error in (no error)"=w402, "PWM Ref In"=w403) -> ()  [unwired: 9 in, 1 out]
      n160 = call <vilib>:"Close.vi"("error in (no error)"=w397, "PWM Ref In"=w404) -> ()  [unwired: 9 in, 1 out]
      n161 = call <vilib>:"Close.vi"("error in (no error)"=w396, "PWM Ref In"=w401) -> ()  [unwired: 9 in, 1 out]
      n162 = call <vilib>:"Close.vi"("error in (no error)"=w395, "PWM Ref In"=w400) -> ()  [unwired: 9 in, 1 out]
      n163 = call <vilib>:"Close.vi"("error in (no error)"=w394, "PWM Ref In"=w399) -> ()  [unwired: 9 in, 1 out]
    }
  }
  n164 = Multiply(x=4.0, y=6.283185307179586) -> (x*y=w5:dbl)
  n165 = Divide(x=w5, y=9600.0) -> (x/y=→"cout per foot":dbl)
